vi "Test String Omnibus Event.vi"() -> ()   [LabVIEW 2021]
uses:
  Source/Omni-Bus/Omni_Bus.lvclass
  Source/Event Bus/Event_Bus.lvclass
  C:/TSA/Omni-Bus/Source/Omni-Bus/Bus Access/Bus_Access.lvclass
  Source/Local Bus/Local Bus.lvclass
  Source/Local Bus/Support/Tag List Type.ctl
  <vilib>/Utility/Data Type/Type Definitions/Data Type.ctl
  <vilib>/TSA/Abstract Data Classes/Abs_Types/Type/Abs_Type.lvclass/Abs_Type.ctl
  Source/Omni-Bus/Omni_Bus.lvclass/Omni_Bus.ctl
  Source/Omni-Bus/Support/Write/Write String.vi
  Source/Omni-Bus/Support/Read/Read String.vi
  Source/Omni-Bus/Support/FindVar.vi
  <vilib>/Utility/error.llb/Clear Errors.vi
  Source/Omni-Bus/Properties/Read Var Map.vi
  <vilib>/TSA/Abstract Data Classes/Abs_Types/Type/Properties/Read Tag.vi
  <vilib>/TSA/Abstract Data Classes/Abs_Types/String/Abs_String.lvclass
  C:/Program Files (x86)/National Instruments/LabVIEW 2021/vi.lib/TSA/Abstract Data Classes/Abs_Types/Type/Abs_Type.lvclass
  <vilib>/TSA/Abstract Data Classes/Abs_Types/Value/Abs_Value.lvclass
  Source/Omni-Bus/Support/Check For Read Only Error.vi
  Source/Omni-Bus/Support/Incorrect Tag String Error.vi
  <vilib>/TSA/Abstract Data Classes/Abs_Types/Type/Abs_Type.lvclass
  <vilib>/Utility/Data Type/NI_Data Type.lvlib
  Source/Omni-Bus/Support/Broad Types.ctl
  C:/TSA/Omni-Bus/Source/Local Bus/Local Bus.lvclass
  C:/TSA/Omni-Bus/Source/Event Bus/Event_Bus.lvclass
panel:
  in  "Combo Box 3":string(combo)
  in  "Combo Box 2":string(combo)
  in  "Combo Box":string(combo)
  in  "stop 6":bool
  out "Numeric 6":i32
  in  "String":string
  out "String 3":string
  in  "String 2":string
  out "Numeric 2":i32
  out "Numeric":i32
  in  "stop 2":bool
  in  "stop":bool
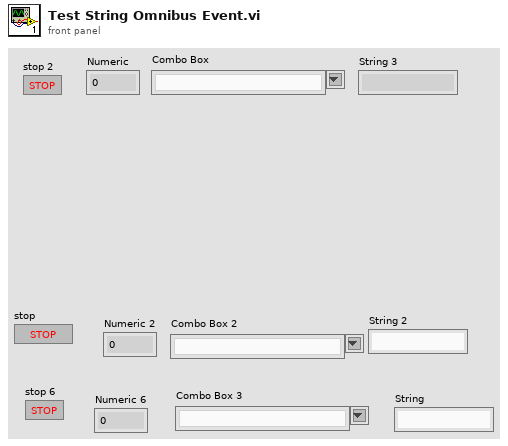
[diagram p1: front panel]
types:
  T1 = typedef "Omni_Bus.lvclass/Broad Types.ctl" = enum16{"All Tags", "NI Specific Type", "Boolean", "String", "Numeric", "Float", "Integer", "Collection", "All Value Types", "Non Value Types"}
  T2 = typedef "Local Bus.lvclass/Tag List Type.ctl" = cluster{"Tag":string, "Type":T3}
  T3 = typedef "NI_Data Type.lvlib/Data Type.ctl" = enum8{"Invalid Type", "Void", "I8", "I16", "I32", "I64", "U8", "U16", "U32", "U64", "Single Float", "Double Float", "Extended Float", "Single Complex", "Double Complex", "Extended Complex", "Enum U8", "Enum U16", "Enum U32", "Enum U64", "Single Float With Unit", "Double Float With Unit", "Extended Float With Unit", "Single Complex with Unit", "Double Complex with Unit", "Extended Complex with Unit", "Boolean", "String", "Path", "Picture", "Tag", "Array", "Cluster", "Variant", "LV Variant", "Waveform", "Timestamp", "Digital Waveform", "Digital Data", "ExpressData", "Refnum", "External Data", "VI", "Poly VI", "LabVIEW Class Instance", "Fixed Point", "Set Collection", "Map Collection"}
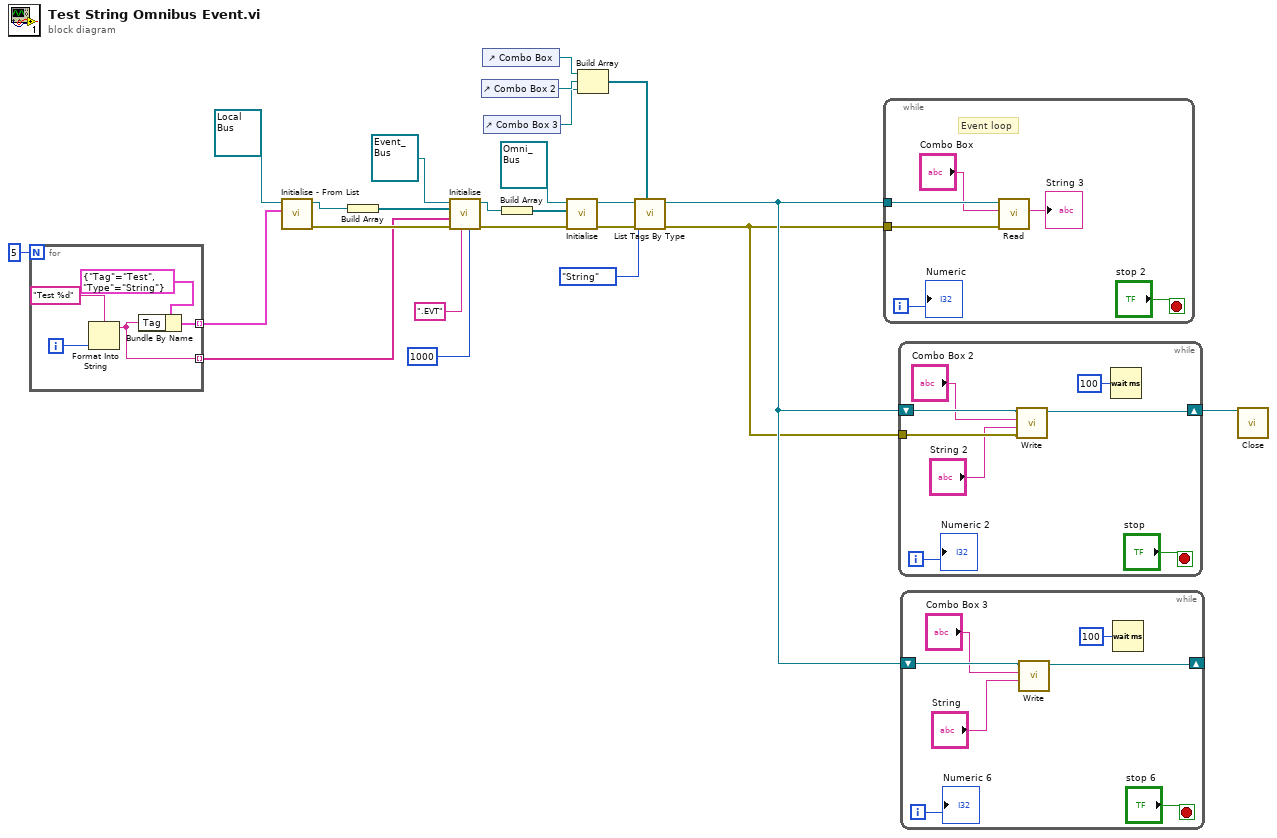
[diagram p0: block diagram]
diagram:
  n1 = for {
    N: 5 -> [_]
    tunnel: [w26] -> w13 mode=indexing
    tunnel: [w25] -> w10 mode=indexing
    i -> [w27]
    n2 = Format Into String(format string="Test %d", w27) -> (resulting string=w25:string)  [unwired: 2 in, 1 out]
    n3 = Bundle By Name(cluster=T2 {"Tag"="Test", "Type"=enum."String"} ("Cluster"), "Tag"=w25) -> (w26:T2)
  }
  n4 = call "Initialise - From List.vi"("Tag List"=w13, "Local Bus in"=refnum<class "Local Bus.lvclass"> refnum) -> ("error out"=w18:errorcluster, "Local Bus out"=w17:refnum<class "Local Bus.lvclass">)  [unwired: 8 in]
  n5 = Build Array(w17) -> (w19:refnum<class "Local Bus.lvclass">[])
  n6 = call "Initialise.vi"("Default Timeout (ms)"=1000, "Tag Root"=".EVT", "error in (no error)"=w18, "Tags to Create Events For"=w10, "Buses"=w19, "Event_Bus in"=refnum<class "Event_Bus.lvclass"> refnum) -> ("error out"=w22:errorcluster, "Event_Bus out"=w21:refnum<class "Event_Bus.lvclass">)  [unwired: 4 in]
  n7 = control-ref of="Combo Box 2"() -> (w4:refnum<vi>)
  n8 = control-ref of="Combo Box"() -> (w5:refnum<vi>)
  n9 = control-ref of="Combo Box 3"() -> (w3:refnum<vi>)
  n10 = Build Array(w21) -> (w23:refnum<class "Event_Bus.lvclass">[])
  n11 = call-dynamic "Initialise.vi"("error in (no error)"=w22, "Bus Access"=w23, "Var Bus in"=refnum<class "Omni_Bus.lvclass"> refnum) -> ("error out"=w7:errorcluster, "Var Bus out"=w9:refnum<class "Omni_Bus.lvclass">)  [unwired: 7 in]
  n12 = Build Array(w5, w4, w3) -> (w2:refnum<vi>[])
  n13 = call "List Tags By Type.vi"("Combo Boxes"=w2, "error in (no error)"=w7, "Broad Types"=Broad_Types."String", "Var Bus in"=w9) -> ("error out"=w6:errorcluster, "Var Bus out"=w8:refnum<class "Omni_Bus.lvclass">)  [unwired: 4 in, 2 out]
  n14 = while {
    tunnel: w8 -> [w35]
    tunnel: w6 -> [w34]
    i -> [w32]
    stop <- "stop 2" stop-if-true
    # "Event loop"
    n15 = call-poly "Read.vi"("error in (no error)"=w34, "Tag"="Combo Box", "Var Bus in"=w35) -> ("String"=→"String 3":string)  [unwired: 6 in, 2 out]
    "Numeric" <- w32
  }
  n16 = while {
    tunnel: w6 -> [w41]
    shift-right: [w38] -> w15
    shift-left: w8 -> [w42]
    i -> [w40]
    stop <- "stop" stop-if-true
    n17 = call-poly "Write.vi"("error in (no error)"=w41, "String"="String 2", "Tag"="Combo Box 2", "Omni_Bus in"=w42) -> ("Omni_Bus out"=w38:refnum<class "Omni_Bus.lvclass">)  [unwired: 6 in, 1 out]
    n18 = Wait (ms)(milliseconds to wait=u32 100) -> ()  [unwired: 1 out]
    "Numeric 2" <- w40
  }
  n19 = while {
    shift-right: [w46] -> _
    shift-left: w8 -> [w49]
    i -> [w48]
    stop <- "stop 6" stop-if-true
    n20 = call-poly "Write.vi"("String"="String", "Tag"="Combo Box 3", "Omni_Bus in"=w49) -> ("Omni_Bus out"=w46:refnum<class "Omni_Bus.lvclass">)  [unwired: 7 in, 1 out]
    n21 = Wait (ms)(milliseconds to wait=u32 100) -> ()  [unwired: 1 out]
    "Numeric 6" <- w48
  }
  n22 = call-dynamic "Close.vi"("Data in"=w15) -> ()  [unwired: 9 in, 2 out]
